vi "currentCOntrolONly.vi"   [LabVIEW 2020]
uses:
  <vilib>/FPGAPlugInAG/cRIO-9054/niLvFpga_Open_cRIO-9054.vi
  <vilib>/rvi/interface/common/dynamic/niFpgaDynamicAddResources.vi
  <vilib>/Utility/error.llb/Error Cluster From Error Code.vi
  <vilib>/rvi/errors/niLvFpgaAdjustHostInterfaceError.vi
  <vilib>/FPGAPlugInAG/Dynamic/niLvFpga_Close_Dynamic.vi
  <vilib>/rvi/interface/nirviOpenFPGA/nirviOpenFPGA.xnode
  FPGA Bitfiles/ver0.1_FPGATarget_FPGAcontrolledVI_cWk4O34ijhk.lvbitx
  FPGA_controlled VI.vi
  <vilib>/rvi/interface/nirviReadWriteControl/nirviReadWriteControl.xnode
  <vilib>/rvi/interface/nirviCloseFPGA/nirviCloseFPGA.xnode
  NiFpgaLv.dll
  <vilib>/rvi/interface/Simulation/niFpgaSimulationCallBeginRW.vi
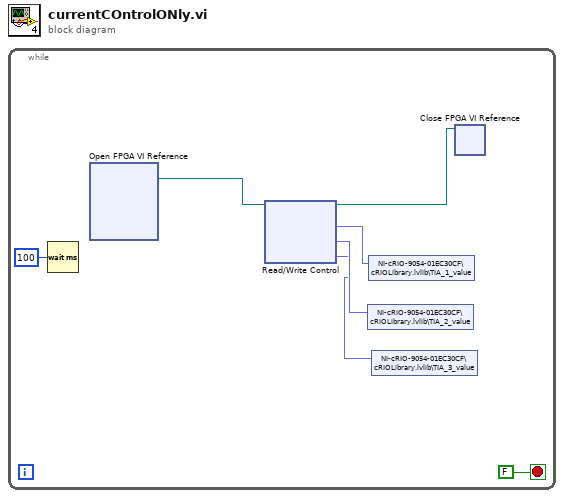
[diagram p0: block diagram]
diagram:
  n1 = while {
    stop <- FALSE stop-if-true
    n2 = Wait (ms)(milliseconds to wait=u32 100) -> ()  [unwired: 1 out]
    n3 = xnode "Open FPGA VI Reference"() -> ("FPGA VI Reference Out"=w7:refnum<k20>)  [unwired: 2 in, 1 out]
    n4 = xnode "Read/Write Control"("FPGA VI Reference In"=w7) -> ("FPGA VI Reference Out"=w6:refnum<k20>, "Mod1/AI7"=w5:fxp<+/-,26,5>, "Mod1/AI8"=w4:fxp<+/-,26,5>, "Mod1/AI9"=w3:fxp<+/-,26,5>)  [unwired: 1 in, 1 out]
    n5 = shared-variable "NI-cRIO-9054-01EC30CF\\cRIOLibrary.lvlib\\TIA_2_value"(w4) -> ()  [unwired: 1 in, 1 out]
    n6 = shared-variable "NI-cRIO-9054-01EC30CF\\cRIOLibrary.lvlib\\TIA_1_value"(w5) -> ()  [unwired: 1 in, 1 out]
    n7 = shared-variable "NI-cRIO-9054-01EC30CF\\cRIOLibrary.lvlib\\TIA_3_value"(w3) -> ()  [unwired: 1 in, 1 out]
    n8 = xnode "Close FPGA VI Reference"("FPGA VI Reference In"=w6) -> ()  [unwired: 1 in, 1 out]
  }
